vi "SamplePath.vi"(11 "Refnum in":refnum<k21>) -> ()   [LabVIEW 2013]
uses:
  <resource>/objmgr/Canvas2D.rc
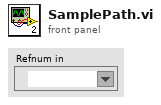
[diagram p1: front panel]
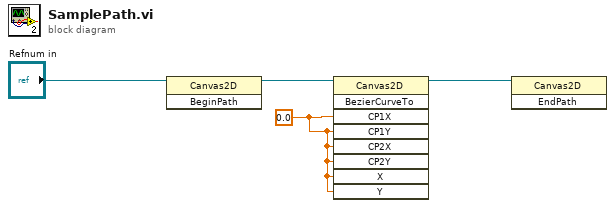
[diagram p0: block diagram]
diagram:
  w1 = 0.0 ("CP1X")
  n1 = invoke class="Canvas2D" method="BeginPath"(reference="Refnum in") -> (reference out=w3:refnum<k21>)  [unwired: 2 in, 2 out]
  n2 = invoke class="Canvas2D" method="BezierCurveTo"(reference=w3, "CP1X"=w1, "CP1Y"=w1, "CP2X"=w1, "CP2Y"=w1, "X"=w1, "Y"=w1) -> (reference out=w2:refnum<k21>)  [unwired: 2 in, 8 out]
  n3 = invoke class="Canvas2D" method="EndPath"(reference=w2) -> ()  [unwired: 2 in, 3 out]
